vi "ILABW_DisplayStatus.vi"() -> ()   [LabVIEW 2012]
panel:
  out "errorOut":string
  in  "time":string
  in  "message":string
  in  "viName":string
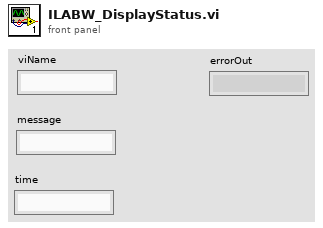
[diagram p1: front panel]
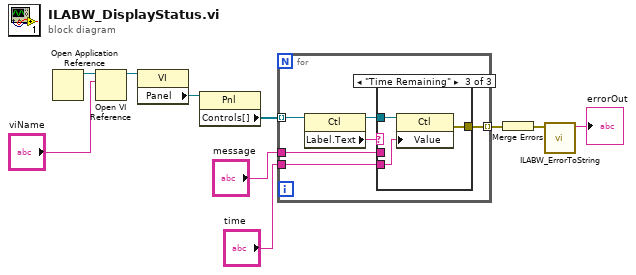
[diagram p0: block diagram]
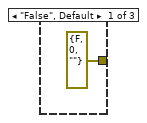
[diagram p2: hidden frame]
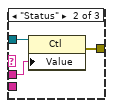
[diagram p3: hidden frame]
diagram:
  n1 = Open Application Reference() -> (3:w9:refnum<vi>)  [unwired: 4 in, 1 out]
  n2 = Open VI Reference(application reference (local)=w9, vi path="viName") -> (vi reference=w8:refnum<vi>)  [unwired: 4 in, 1 out]
  n3 = property class="VI"(reference=w8) -> ("Panel"=w7:refnum<vi>)  [unwired: 1 in, 2 out]
  n4 = property class="Pnl"(reference=w7) -> ("Controls[]"=w6:refnum<vi>[])  [unwired: 1 in, 2 out]
  n5 = for {
    tunnel: w6 -> [w16] mode=indexing
    tunnel: "message" -> [w13]
    tunnel: [w12] -> w3 mode=indexing
    tunnel: "time" -> [w11]
    n6 = property class="Ctl"(reference=w16) -> (reference out=w14:refnum<vi>, "Label.Text"=w15:string)  [unwired: 1 in, 1 out]
    n7 = case shown="\"Time Remaining\"" w15 {
      tunnel: w14 -> [_ w20 w23]
      tunnel: w13 -> [_ w19 _]
      tunnel: [errorcluster {"status"=FALSE, "code"=0, "source"=""} ("error out") w18 w21] -> w12
      tunnel: w11 -> [_ _ w22]
      frame "False", Default {
      }
      frame "Status" {
        n8 = property class="Ctl"(reference=w20, "Value"=w19) -> (error out=w18:errorcluster)  [unwired: 1 in, 1 out]
      }
      frame "Time Remaining" {
        n9 = property class="Ctl"(reference=w23, "Value"=w22) -> (error out=w21:errorcluster)  [unwired: 1 in, 1 out]
      }
    }
  }
  n10 = Merge Errors(w3) -> (w2:errorcluster)
  n11 = call "ILABW_ErrorToString.vi"("errorIn"=w2) -> ("errorOut"=→"errorOut":string)  [unwired: 10 in]
